vi "About.vi"(8 "error in (no error)":errorcluster) -> (0 "error out":errorcluster)   [LabVIEW 2015]
uses:
  <vilib>/Platform/browser.llb/Open URL in Default Browser (string).vi
panel:
  in  "Link Text":bool
  in  "OK Button":bool
  in  "Body":string caption="Error description"
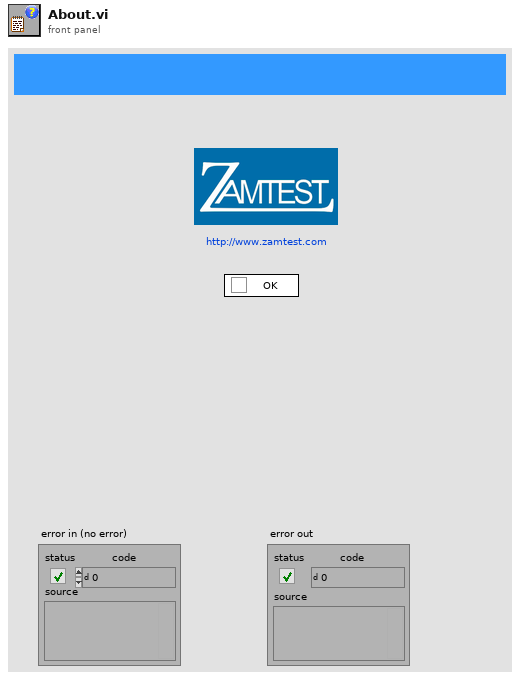
[diagram p1: front panel]
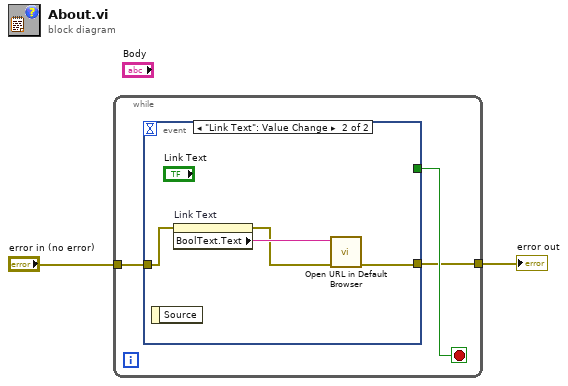
[diagram p0: block diagram]
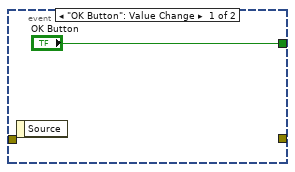
[diagram p2: hidden frame]
diagram:
  n1 = while {
    tunnel: "error in (no error)" -> [w4]
    tunnel: [w3] -> w1
    stop <- w5 stop-if-true
    n2 = event shown="[1] \"Link Text\": Value Change" {
      selector: _ -> [_ _]
      dyn-events: _ -> [_ _]
      timeout: _ -> [_ _]
      tunnel: ["OK Button" _] -> w5
      tunnel: w4 -> [_ w9]
      tunnel: [_ w7] -> w3
      event "OK Button": Value Change {
        n3 = event-data() -> ()  [unwired: 1 in, 1 out]
      }
      event "Link Text": Value Change {
        n4 = event-data() -> ()  [unwired: 1 in, 1 out]
        n5 = property on="Link Text" class="Bool"(error in=w9) -> (error out=w8:errorcluster, "BoolText.Text"=w10:string)  [unwired: 1 in, 1 out]
        n6 = call-poly <vilib>:"Open URL in Default Browser.vi"("error in (no error)"=w8, "URL"=w10) -> ("error out"=w7:errorcluster)  [unwired: 4 in, 1 out]
      }
    }
  }
  "error out" <- w1
